vi "SCCSup Message Strings GLBL.vi"() -> ()   [LabVIEW 2017]
panel:
  in  "P4 filehist diff err":string="Comparing this file type is not supported from this dialog. "
  in  "P4 filehist popup 2":string[](array[string])=["Diff 2 revisions"]
  in  "missfilemsg":string="One or more missing files cannot be retrieved from source code control."
  in  "missing or out of date proj msg":string="The project file is out-of-date or missing. Select Tools>>Source Control>>Get Latest Version to get the latest version of the project file."
  in  "no missing items":string="No items found in project."
  in  "Continue":string="Continue"
  in  "prjlvlscc_connmsg_prjerr_envprj":string="Select %s then click the %s button to reconfigure the environment source control project."
  in  "prjlvlscc_connmsg_prjerr_prj":string="Select another option from above to reconfigure the source control settings for this LabVIEW project."
  in  "prjlvlscc_connmsg_prjerr_env":string="Click the %s button to reconfigure the environment source control project."
  in  "Change":string="Change"
  in  "environment":string="environment"
  in  "Tools_SCC":string="Tools>>Source Control>>Configure Source Control"
  in  "specified":string="specified"
  in  "SourceControlProviderName":string="Source Control Provider Name"
  in  "MAI":string="the main application instance"
  in  "LabVIEWProject":string="this LabVIEW project"
  in  "prjlvlscc_prjsettings_err":string="LabVIEW was unable to open the source control project for %s. The source control settings might not be valid for this session or a timeout occurred. Source control will not be available in %s.\n\nSelect Tools>>Source Control>>Configure Source Control or Project>>Properties  to reconfigure source control.\n\nAdditional Information:\n%s"
  in  "prjlvlscc_switchtoenv":string="LabVIEW was unable to open the default source control project. Using this setting will result in source control not being available for this LabVIEW project.\n\nDo you want to proceed?\n\n"
  in  "prjlvlscc_connmsg_prjerr":string="Source control is currently unavailable for %s.  LabVIEW was unable to open the %s source control project.\n\n%s"
  in  "prjlvlscc_connmsg_enverr":string="Source control is currently unavailable in LabVIEW. LabVIEW was unable to connect to the specified source control provider (%s).\n\nSelect %s then select a provider from the %s pull-down menu to reconfigure source control in LabVIEW."
  in  "prjlvlscc_connmsg_conflict":string="Source control is currently unavailable for %s. This LabVIEW project's source control settings conflict with the LabVIEW environment settings. The source control project settings require %s.\n\nSelect %s to change the source control provider in LabVIEW."
  in  "prjlvlscc_connmsg_noscccfg":string="%s\n\nSelect %s to enable source control in LabVIEW."
  in  "prjlvlscc_noscccfg":string="No source control provider is configured."
  in  "prjlvlscc_envmsg":string="The configured source control provider is %s.\n\nSelect %s to change the environment source control settings."
  in  "unsaved sccop msg":string="You need to save these files before performing the source control operation.\n\nDo you want to save these files now?"
  in  "unsaved checkin msg":string="The following files have unsaved changes. \n\nWould you like to save these files before checking them into source control?"
  in  "intro screen msg":string="Version %s (%s-bit) - Connecting to %s"
  in  "no files for op":string="The selected files' source control status is not valid for this operation."
  in  "continue checkin prompt":string="You chose not to save the file(s) with unsaved changes. If you proceed with the check in operation, the most recently saved file(s) on disk will be checked in. Unsaved changes will not be reflected in the checked in files.\n\nDo you want to proceed with the check in operation?"
  in  "P4 filehist popup":string[](array[string])=["Sync to this revision", "Describe changelist"]
  in  "P4 file identical":string="%s does not differ from the depot version."
  in  "check out warning":string="Checking out this file will also check out the files of all callers that are in memory.\n\nRefer to the Source Control Options Page of the LabVIEW Help for more information about including callers when checking out files.\n\nDo you want to proceed?"
  in  "connection dialog msg":string="Connecting to %s ..."
  in  "connect prob msg":string="Source control is currently unavailable in LabVIEW. LabVIEW was unable to connect to the specified source control provider (%s).\n\nSelect a provider from the %s pull-down menu to reconfigure source control in LabVIEW."
  in  "undochkout warning":string="The source control provider's version of the specified files will be copied to your computer. Any changes made in your copies of these files will be lost.\n\nDo you want to proceed?"
  in  "multiple items selected":string="(multiple items selected)"
  in  "no category name":string="Generic Item"
  in  "Dependents":string="Dependents"
  in  "Callers":string="Callers"
  in  "Cancel":string="Cancel"
  in  "OK":string="OK"
  in  "add to SCC prompt":string="The following file(s) are currently not in source control:\n\n%s\n\nDo you want to add the file(s) to source control?"
  in  "server access warning":string="LabVIEW could not access the %s server. The LabVIEW configuration settings might not be valid for this session or a timeout occurred. Source control will not be available in LabVIEW.\n\nSelect Tools>>Options to reconfigure source control.\n\nAdditional Information:\n%s"
  in  "edit on chkout prompt":string="You are modifying the following file(s):\n\n%s\n\nThe file(s) have not been checked out of source control. Do you want to check the file(s) out?"
  in  "remove warning":string="The source control provider will remove the specified files on its server. The local copies may or may not be deleted depending on the provider's configuration. If local copies are deleted, any changes in opened copies of the selected files will be lost when they are closed.\n\nDo you want to proceed?"
  in  "get latest warning":string="The source control provider's latest version of the specified files will be copied to your computer. Any changes made in these file will be lost. To view the retrieved versions, you may need to close any opened files then reload them.\n\nDo you want to proceed?"
  in  "Tools":string="Tools"
  in  "add unsaved VIs msg":string="You cannot add an unsaved file to source control.\n\nPlease save the file(s) and then try the add operation again. "
  in  "scc toolbar desc":string[](array[string])=["Check Out", "Undo Check Out", "Check In", "", "Add to Source Control"]
  in  "scc prj menu entries":string[](array[string])=["Get Latest Version...", "Check In...", "Check Out", "Undo Check Out...", "", "Add to Source Control...", "Remove from Source Control...", "", "Show History...", "Show Differences...", "Properties...", "Refresh Status", "", "Run %s Client...", "", "Configure Source Control...", "Get Latest Version of All Files..."]
  in  "other out message":string="The following file(s) are checked out by another user:\n\n%s\n\nDo you want to check the file(s) out?"
  in  "no":string="No"
  in  "yes":string="Yes"
  in  "cancel prov change":string="Are you sure you want to cancel source control project configuration?  If you cancel, the current source control project configuration will be used."
  in  "P4 verfile chnglist msg":string="The following file(s) are not in changelist \"%s\":\n%s"
  in  "P4 verfile prob msg":string="The following file(s) had problems:\n%s"
  in  "P4 submit bad desc msg":string="Please enter a valid description."
  in  "P4 filehist dlg title":string="Perforce Revision History for %s"
  in  "P4 filehist colhead":string[](array[string])=["Revision", "Changelist", "Date", "User", "Action"]
  in  "P4 show only clients":string="Only show clients containing \"%s\""
  in  "P4 select client":string="Select Client Workspace"
  in  "P4 browse clients colhead":string[](array[string])=["Client", "Mod Date", "Client Root", "Description"]
  in  "P4 select user":string="Select User"
  in  "P4 browse users colhead":string[](array[string])=["User", "Email", "Full Name", "Access Time"]
  in  "P4 paths msg":string="Perforce must be installed in one of the following paths:\n"
  in  "P4 cancel sync msg":string="User cancellation of sync operation."
  in  "P4 sync during chkout msg":string="The following file(s) are out of date:\n\n%s\n\nSync all to head revision before editing?"
  in  "P4 notice title":string="Perforce Notice"
  in  "getprojopts":string="get the source control project options."
  in  "copy msg":string="copy the specified file."
  in  "cfg  no prov":string="You have selected not to use any source control provider.\n\nLabVIEW will disconnect from the current provider.  Continue?"
  in  "cfg  prov change":string="The provider name has been changed.\n\nChanging to a different provider can cause unexpected behavior.\nContinue?"
  in  "none":string="< None >"
  in  "dialog title":string[](array[string])=["Get Latest Version", "Check Out File(s)", "Check In File(s)", "Undo Check Out", "Add to Source Control", "Remove from Source Control"]
  in  "op msg":string="An error occurred trying to "
  in  "provider msg":string="The source control provider returned the following information:"
  in  "SourceControl":string="Source Control"
  in  "undocheckout msg":string="undo the check out the specified file(s)."
  in  "runscc msg":string="run the source code provider's administration tool."
  in  "rename msg":string="rename the specified file."
  in  "remove msg":string="remove the specified file(s) from source control."
  in  "query msg":string="access the status of the specified file(s)."
  in  "suppfunc msg":string="access the functionality of the source control provider."
  in  "suppadvcmd msg":string="verify if source control provider supports advanced command options."
  in  "openproj msg":string="create or open a source control project."
  in  "getprojpath msg":string="get the source control project path."
  in  "getlatest msg":string="get the specified file(s)."
  in  "disconnect msg":string="disconnect from the source control provider."
  in  "checkout msg":string="check out the specified file(s)."
  in  "checkin msg":string="check in the specified file(s)."
  in  "add msg":string="add the specified file(s) to the source control system."
  in  "getcmdopt msg":string="get advanced options for a command."
  in  "history msg":string="access the history of the specified file(s)."
  in  "properties msg":string="display the properties of the specified file(s)."
  in  "uninit msg":string="uninitialize the source control provider."
  in  "connect msg":string="connect to the source control provider (%s)."
  in  "compare msg":string="compare the specified file with the most recently checked in version."
  # "provider and config dialog strings"
  # "perforce command line"
  # "Error strings"
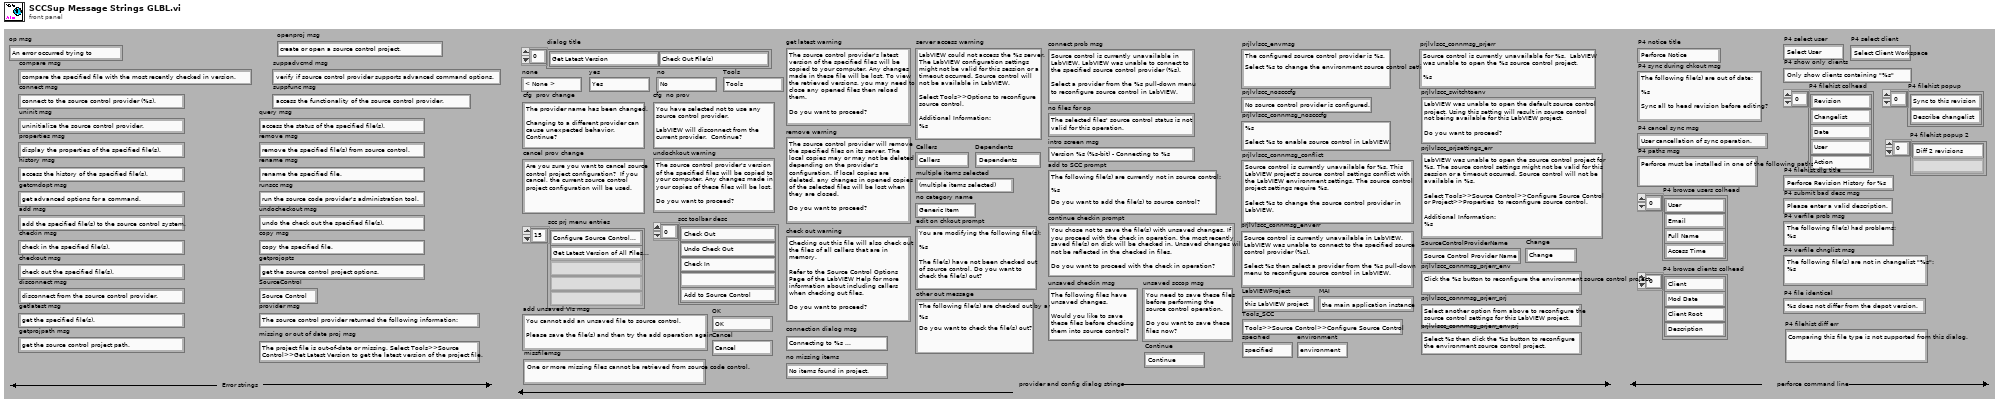
[diagram p1: front panel]
diagram:
